vi "Get Boolean.vi"(8 "error in (no error)":errorcluster, 9 "Data Type (default value)":bool, 10 "Offset":i32, 11 "JSON":string) -> (0 "error out":errorcluster, 1 "Boolean":bool, 2 "Offset past match":i32)   [LabVIEW 2017, in "JSONtext.lvlib"]
uses:
  JSONtext.lvlib
  <vilib>/Utility/error.llb/Error Cluster From Error Code.vi
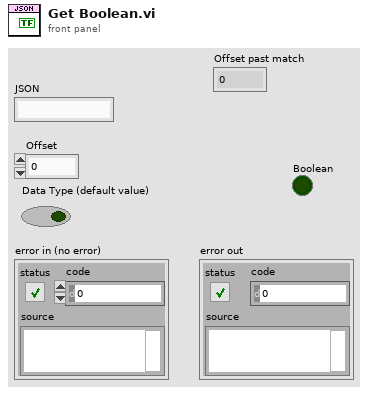
[diagram p1: front panel]
types:
  T1 = typedef "JSONtext.lvlib/Parsing State.ctl" = enum16{"Parser Error", "Object", "Array", "String", "Number/Other", "Leading Whitespace", "Object end", "Array end", "Value end"}
  T2 = typedef "JSONtext.lvlib/JSON Value Type.ctl" = enum16{"Not a JSON Value", "JSON Object", "JSON Array", "String", "Number", "true", "false", "null"}
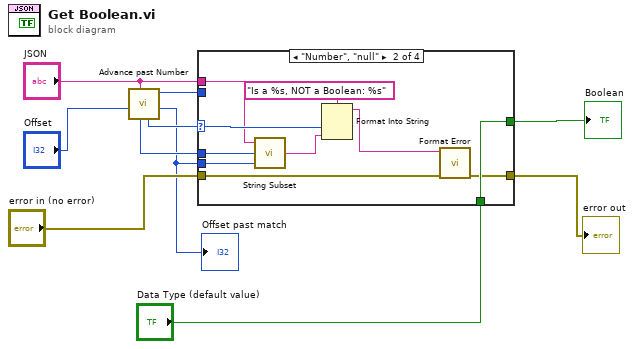
[diagram p0: block diagram]
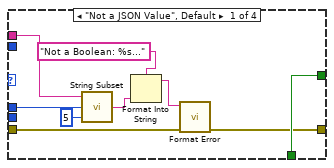
[diagram p2: hidden frame]
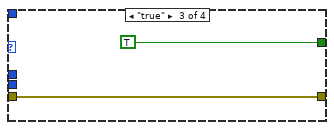
[diagram p3: hidden frame]
diagram:
  n1 = call "Advance past Number.vi"("JSON"="JSON", "Offset (0)"="Offset") -> ("Offset past match"=w3:i32, "Parser State"=w1:T1, "JSON Value Type"=w6:T2, "Value start out"=w4:i32)  [unwired: 6 in]
  "Offset past match" <- w3
  n2 = case shown="\"Number\", \"null\"" w6 {
    selector: w6 -> [_ w26 _ _]
    tunnel: [w19 w29 TRUE _] -> w10
    tunnel: [w18 w28 w30 w32] -> w9
    tunnel: "error in (no error)" -> [w17 w27 w30 w32]
    tunnel: "Data Type (default value)" -> [w19 w29 _ _]
    tunnel: w4 -> [w15 w23 _ _]
    tunnel: w3 -> [_ w22 _ _]
    tunnel: "JSON" -> [w16 w21 _ _]
    tunnel: w1 -> [_ _ _ _]
    frame "Not a JSON Value", Default {
      n3 = call "String Subset.vi"("Offset past End"=5, "Start offset"=w15, "JSON"=w16) -> ("substring"=w12:string)  [unwired: 2 in]
      n4 = Format Into String(format string="Not a Boolean: %s...", w12) -> (resulting string=w11:string)  [unwired: 2 in, 1 out]
      n5 = call "Format Error.vi"("error in (no error)"=w17, "error message"=w11) -> ("error out"=w18:errorcluster)  [unwired: 9 in]
    }
    frame "Number", "null" {
      n6 = call "String Subset.vi"("Offset past End"=w22, "Start offset"=w23, "JSON"=w21) -> ("substring"=w20:string)  [unwired: 2 in]
      n7 = Format Into String(format string="Is a %s, NOT a Boolean: %s", w26, w20) -> (resulting string=w24:string)  [unwired: 2 in, 1 out]
      n8 = call "Format Error.vi"("error in (no error)"=w27, "error message"=w24) -> ("error out"=w28:errorcluster)  [unwired: 9 in]
    }
    frame "true" {
    }
    frame "false" {
    }
  }
  "error out" <- w9
  "Boolean" <- w10
